vi "solar_qtimer Destroy2.vi"(6 "Suppress Errors? (T)":bool=TRUE, 8 "error in (no error)":errorcluster, 11 "QTimer Refnum":T1) -> (0 "error out":errorcluster)   [LabVIEW 2018]
doc: "This releases the QTimer reference."
uses:
  solar_qtimer_ctl Refnum.ctl
panel:
  out "Array":errorcluster[](array[cluster])
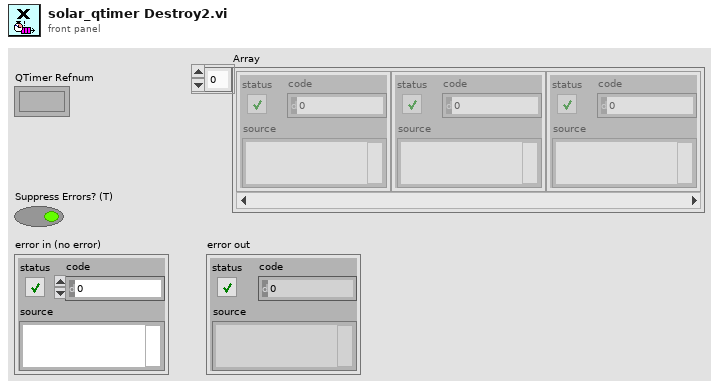
[diagram p1: front panel]
types:
  T1 = typedef "solar_qtimer_ctl Refnum.ctl" = refnum<k1>
  T2 = typedef "solar_qtimer_ctl SEQ.ctl" = cluster{"QTimers":T3[]}
  T3 = typedef "solar_qtimer_ctl QTimer.ctl" = cluster{"Settings":T4, "Queue":refnum<queue>, "QTimerQ":refnum<queue>, "VI Refnum":refnum<vi>}
  T4 = typedef "solar_qtimer_ctl QTimer Settings.ctl" = cluster{"QTimer":string, "Delay":i32, "Start":bool, "EnQ_Type":enum8{"Normal", "Priority", "IgnoreIfExists"}, "Messages":cluster{"MSG":string, "DATA":variant}[]}
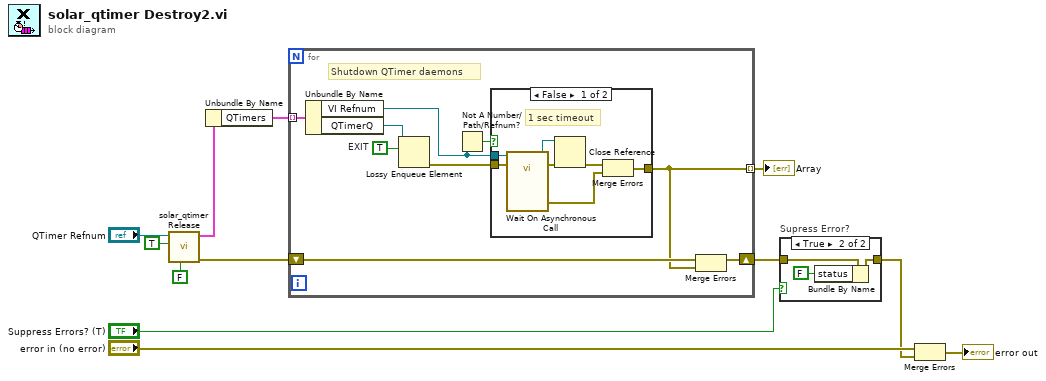
[diagram p0: block diagram]
diagram:
  n1 = call "solar_qtimer Release.vi"("Suppress Errors? (T)"=FALSE, "Force Destroy? (F)"=TRUE, "QTimer Refnum"="QTimer Refnum") -> ("error out"=w4:errorcluster, "QTimer"=w7:T2)  [unwired: 7 in]
  n2 = Unbundle By Name(w7) -> ("QTimers"=w3:T3[])
  n3 = for {
    shift-right: [w19] -> w1
    shift-left: w4 -> [w21]
    tunnel: w3 -> [w20] mode=indexing
    tunnel: [w15] -> w2 mode=indexing
    w17 = TRUE  # EXIT
    # "Shutdown QTimer daemons"
    n4 = Unbundle By Name(w20) -> ("VI Refnum"=w14:refnum<vi>, "QTimerQ"=w18:refnum<queue>)
    n5 = Lossy Enqueue Element(queue=w18, element=w17) -> (error out=w16:errorcluster)  [unwired: 1 in, 3 out]
    n6 = Not A Number/Path/Refnum?(number/path/refnum=w14) -> (NaN/Path/Refnum?=w13:bool)
    n7 = case shown="False" w13 {
      tunnel: w16 -> [w28 w29]
      tunnel: w14 -> [w27 _]
      tunnel: [w22 w29] -> w15
      frame False {
        # "1 sec timeout"
        n8 = call-by-ref "Wait On Asynchronous Call"(reference=w27, error in=w28) -> (reference out=w25:refnum<vi>, error out=w24:errorcluster, "Error"=w26:errorcluster)  [unwired: 11 in]
        n9 = Close Reference(reference=w25, error in (no error)=w24) -> (error out=w23:errorcluster)
        n10 = Merge Errors(w23, w26) -> (w22:errorcluster)
      }
      frame True {
      }
    }
    n11 = Merge Errors(w21, w15) -> (w19:errorcluster)
  }
  "Array" <- w2
  n12 = case "Supress Error?" shown="True" "Suppress Errors? (T)" {
    tunnel: w1 -> [w30 w33]
    tunnel: [w30 w31] -> w5
    frame False {
    }
    frame True {
      n13 = Bundle By Name(cluster=w33, "status"=FALSE) -> (w31:errorcluster)
    }
  }
  n14 = Merge Errors("error in (no error)", w5) -> (→"error out":errorcluster)
